vi "Get or Create Channel Index.vi"(8 "error in (no error)":errorcluster, 10 "Channel Definition":T1 {"Custom Config Data" format="%x"}, 11 "CIFCorePlugin in":refnum<class "CIFCorePlugin.lvclass">) -> (0 "error out":errorcluster, 1 "Created":bool, 2 "Channel Index":i32, 3 "CIFCorePlugin out":refnum<class "CIFCorePlugin.lvclass">)   [LabVIEW 2021, in "CIFCorePlugin.lvclass"]
doc: "Look up the index of a channel by name. If the channel does not exist this will create the channel and return the index. This can be used when channels are determined dynamically at run-time instead of when the plugin is designed so the enum is not an option. Best practice is to save the returned indexes and only perform string operations when the channel list changes."
uses:
  CIFCorePlugin.lvclass
  CIFCorePlugin.lvclass/CIFCorePlugin.ctl
  Channels/ChannelRegistrar/ChannelRegistrar.lvlib
  <vilib>/CIF Foundation/CIF Channels Core/ChannelCommon/typedef/Direction.ctl
  <vilib>/CIF Foundation/CIF Channels Core/ChannelCommon/ChannelCommon.lvlib
  Channels/ChannelRegistrar/typedef/Registered Channel Types.ctl
  Channels/ChannelRegistrar/typedef/Channel Definition.ctl
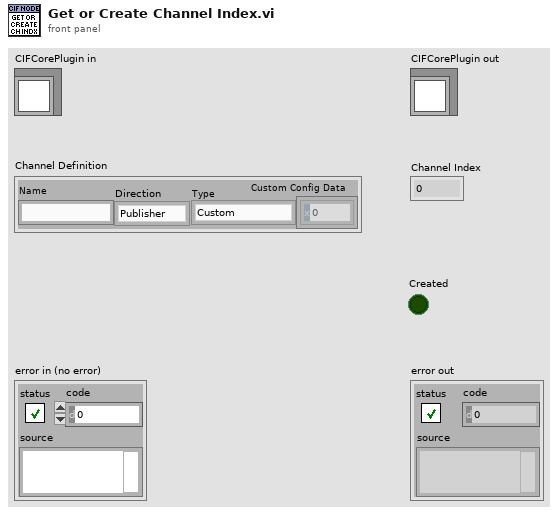
[diagram p1: front panel]
types:
  T1 = typedef "ChannelRegistrar.lvlib/Channel Definition.ctl" = cluster{"Name":string, "Direction":T2, "Type":T3, "Custom Config Data":u8[]}
  T2 = typedef "ChannelCommon.lvlib/Direction.ctl" = enum8{"Publisher", "Subscriber"}
  T3 = typedef "ChannelRegistrar.lvlib/Registered Channel Types.ctl" = enum8{"Custom", "Double_Tag", "I64_Tag", "U64_Tag", "U8_FIFO", "CAN_FIFO", "L2Enet_FIFO", "DAQ_FIFO", "Universal_FIFO", "String_Tag"}
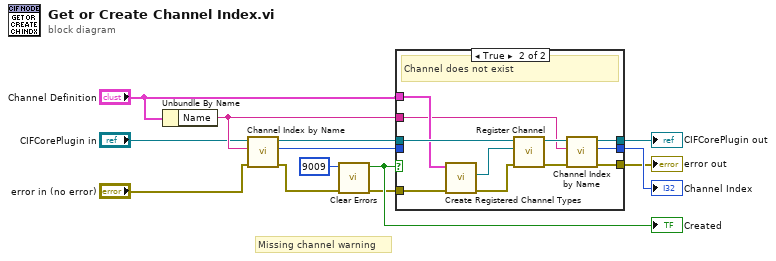
[diagram p0: block diagram]
diagram:
  # "Missing channel warning"
  n1 = Unbundle By Name("Channel Definition") -> ("Name"=w7:string)
  n2 = call "Channel Index by Name.vi"("error in (no error)"="error in (no error)", "Channel Name"=w7, "CIFCorePlugin in"="CIFCorePlugin in") -> ("error out"=w10:errorcluster, "Channel Index"=w12:i32, "CIFCorePlugin out"=w13:refnum<class "CIFCorePlugin.lvclass">)  [unwired: 6 in]
  n3 = call <vilib>:"Clear Errors.vi"("error in (no error)"=w10, "specific error code to clear (0: all)"=9009) -> ("error out"=w8:errorcluster, "specific error cleared?"=w9:bool)  [unwired: 4 in]
  "Created" <- w9
  n4 = case shown="True" w9 {
    tunnel: w13 -> [w16 w27]
    tunnel: w12 -> [w15 _]
    tunnel: w8 -> [w14 w26]
    tunnel: w7 -> [_ w20]
    tunnel: "Channel Definition" -> [_ w23]
    tunnel: [w16 w19] -> w2
    tunnel: [w14 w18] -> w1
    tunnel: [w15 w17] -> w5
    frame False {
      # "Channel exists"
    }
    frame True {
      # "Channel does not exist"
      n5 = call "Create Registered Channel Types.vi"("error in"=w26, "Channel Definition in"=w23) -> ("error out"=w25:errorcluster, "Channel out"=w24:refnum<class "CIFChannels.lvclass">)  [unwired: 6 in, 2 out]
      n6 = call "Register Channel.vi"("error in (no error)"=w25, "Channel"=w24, "CIFCorePlugin in"=w27) -> ("error out"=w21:errorcluster, "CIFCorePlugin out"=w22:refnum<class "CIFCorePlugin.lvclass">)  [unwired: 7 in]
      n7 = call "Channel Index by Name.vi"("error in (no error)"=w21, "Channel Name"=w20, "CIFCorePlugin in"=w22) -> ("error out"=w18:errorcluster, "Channel Index"=w17:i32, "CIFCorePlugin out"=w19:refnum<class "CIFCorePlugin.lvclass">)  [unwired: 6 in]
    }
  }
  "error out" <- w1
  "CIFCorePlugin out" <- w2
  "Channel Index" <- w5
